vi "CheckFoldExit_CreatFold.vi"(0 "path in":path, 1 "FoldOrFile¡H":bool) -> (2 "File out":path, 3 "Fold out":path, 4 "file or folder exists?":bool caption="文件或文件夹存在？")   [LabVIEW 2014]
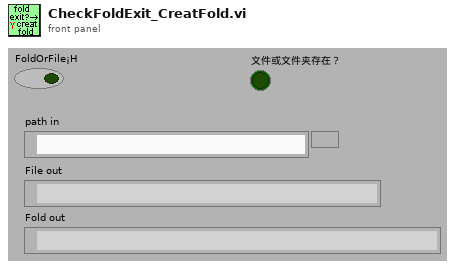
[diagram p1: front panel]
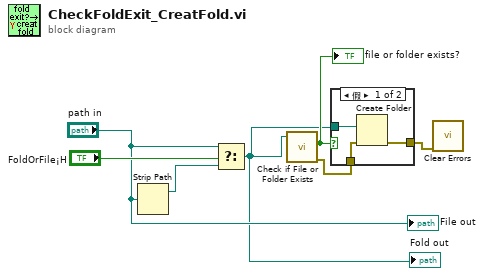
[diagram p0: block diagram]
diagram:
  n1 = Strip Path(path="path in") -> (stripped path=w5:path)  [unwired: 1 out]
  n2 = Select(t="path in", s="FoldOrFile¡H", f=w5) -> (s? t:f=w3:path)
  "Fold out" <- w3
  n3 = call <vilib>:"Check if File or Folder Exists.vi"("path"=w3) -> ("error out"=w2:errorcluster, "file or folder exists?"=w7:bool)  [unwired: 1 in, 8 out]
  "file or folder exists?" <- w7
  n4 = case shown="假" w7 {
    tunnel: w3 -> [w10 _]
    tunnel: w2 -> [w9 w11]
    tunnel: [w8 w11] -> w1
    frame False {
      n5 = Create Folder(path (use dialog)=w10, error in=w9) -> (error out=w8:errorcluster)  [unwired: 3 out]
    }
    frame True {
    }
  }
  n6 = call <vilib>:"Clear Errors.vi"("error in (no error)"=w1) -> ()  [unwired: 5 in, 2 out]
  "File out" <- "path in"
